vi "ConsumeWhitespace.vi"(8 "error in (no error)":errorcluster, 11 "TransformTokenizer in":refnum<class "TransformTokenizer.lvclass">) -> (0 "error out":errorcluster, 3 "TransformTokenizer out":refnum<class "TransformTokenizer.lvclass">)   [LabVIEW 2019, in "TransformTokenizer.lvclass"]
uses:
  TransformTokenizer.lvclass
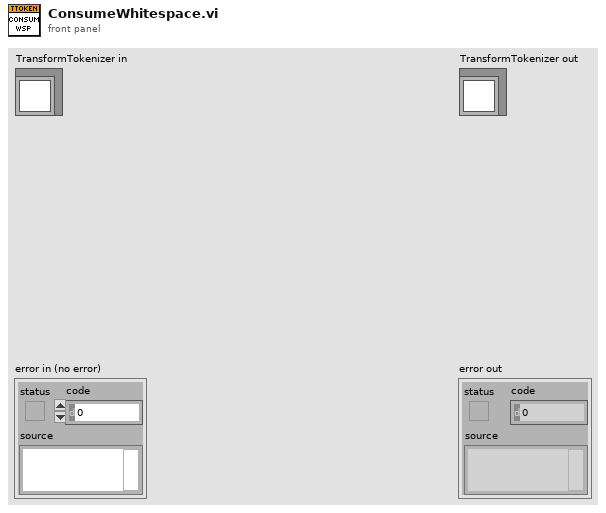
[diagram p1: front panel]
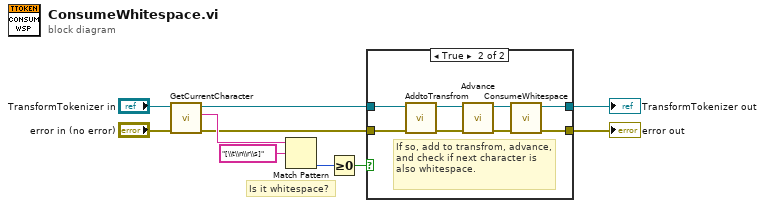
[diagram p0: block diagram]
diagram:
  # "Is it whitespace?"
  n1 = call "GetCurrentCharacter.vi"("error in (no error)"="error in (no error)", "TransformTokenizer in"="TransformTokenizer in") -> ("error out"=w2:errorcluster, "Character"=w3:string, "TransformTokenizer out"=w6:refnum<class "TransformTokenizer.lvclass">)  [unwired: 7 in]
  n2 = Match Pattern(string=w3, regular expression="[\\t\\n\\r\\s]") -> (offset past match=w7:i32)  [unwired: 1 in, 3 out]
  n3 = Greater Or Equal To 0?(x=w7) -> (x >= 0?=w1:bool)
  n4 = case shown="True" w1 {
    tunnel: w6 -> [w11 w15]
    tunnel: [w11 w19] -> w5
    tunnel: w2 -> [w12 w13]
    tunnel: [w12 w17] -> w4
    frame False {
    }
    frame True {
      # "If so, add to transfrom, advance, and check if next character is also whitespace."
      n5 = call "AddtoTransfrom.vi"("error in (no error)"=w13, "TransformTokenizer in"=w15) -> ("error out"=w14:errorcluster, "TransformTokenizer out"=w16:refnum<class "TransformTokenizer.lvclass">)  [unwired: 8 in]
      n6 = call "Advance.vi"("error in (no error)"=w14, "TransformTokenizer in"=w16) -> ("error out"=w18:errorcluster, "TransformTokenizer out"=w20:refnum<class "TransformTokenizer.lvclass">)  [unwired: 8 in]
      n7 = call "ConsumeWhitespace.vi"("error in (no error)"=w18, "TransformTokenizer in"=w20) -> ("error out"=w17:errorcluster, "TransformTokenizer out"=w19:refnum<class "TransformTokenizer.lvclass">)  [unwired: 8 in]
    }
  }
  "error out" <- w4
  "TransformTokenizer out" <- w5
